vi "pulsePIP.vi"(8 "error in (no error)":errorcluster) -> (0 "error out":errorcluster, 3 "PULSE-17":string)   [LabVIEW 2018]
uses:
  Global_usbComm.vi
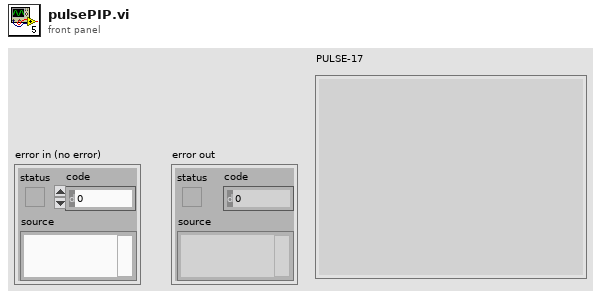
[diagram p1: front panel]
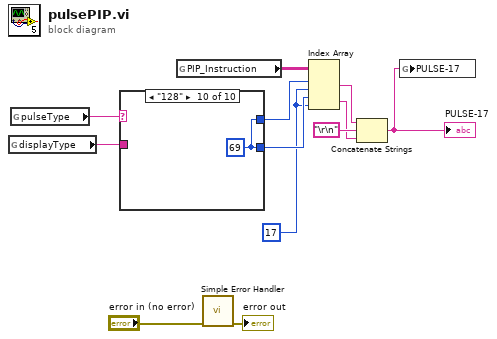
[diagram p0: block diagram]
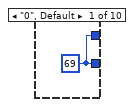
[diagram p2: hidden frame]
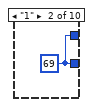
[diagram p3: hidden frame]
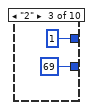
[diagram p4: hidden frame]
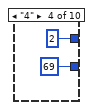
[diagram p5: hidden frame]
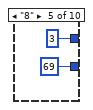
[diagram p6: hidden frame]
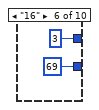
[diagram p7: hidden frame]
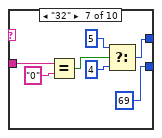
[diagram p8: hidden frame]
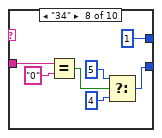
[diagram p9: hidden frame]
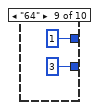
[diagram p10: hidden frame]
diagram:
  w3 = 17
  n1 = global read "Global_usbComm.vi" "displayType"() -> (w10:string)
  n2 = global read "Global_usbComm.vi" "pulseType"() -> (w9:string)
  n3 = case shown="\"128\"" w9 {
    tunnel: [w13 w14 69 69 69 69 69 w33 3 w39] -> w8
    tunnel: [w13 w14 1 2 3 3 w23 1 1 w39] -> w7
    tunnel: w10 -> [_ _ _ _ _ _ w25 w30 _ _]
    frame "0", Default {
      w13 = 69
    }
    frame "1" {
      w14 = 69
    }
    frame "2" {
    }
    frame "4" {
    }
    frame "8" {
    }
    frame "16" {
    }
    frame "32" {
      n4 = Equal?(x=w25, y="0") -> (x = y?=w29:bool)
      n5 = Select(t=5, s=w29, f=4) -> (s? t:f=w23:i32)
    }
    frame "34" {
      n6 = Equal?(x=w30, y="0") -> (x = y?=w36:bool)
      n7 = Select(t=5, s=w36, f=4) -> (s? t:f=w33:i32)
    }
    frame "64" {
    }
    frame "128" {
      w39 = 69
    }
  }
  n8 = global read "Global_usbComm.vi" "PIP_Instruction"() -> (w1:string[][])
  n9 = call <vilib>:"Simple Error Handler.vi"("error in (no error)"="error in (no error)") -> ("error out"=→"error out":errorcluster)  [unwired: 4 in, 4 out]
  n10 = Index Array(array=w1, index (row) #1=w7, index (col) #1=w3, index (row) #2=w8, index (col) #2=w3) -> (element #1=w4:string, element #2=w5:string)
  n11 = Concatenate Strings(w4, "\r\n", w5) -> (w2:string)
  "PULSE-17" <- w2
  n12 = global write "Global_usbComm.vi" "PULSE-17"(w2) -> ()
